vi "identifyPortTypeWithFirstByte_2.vi"(1 "input_str":string) -> (0 "show_str_portType":string)   [LabVIEW 2011]
panel:
  # "本VI已经验证过下列对应关系        OK\nhex  decimal  portType\n03    3           SFP+\n\n11    17          QSFP+\n0D    13         QSFP+\n\n0F     15         HD\n10     16         HD\n14     20         HD\n15     21         HD"
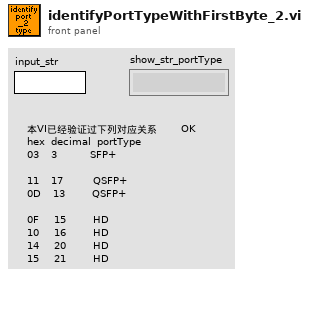
[diagram p1: front panel]
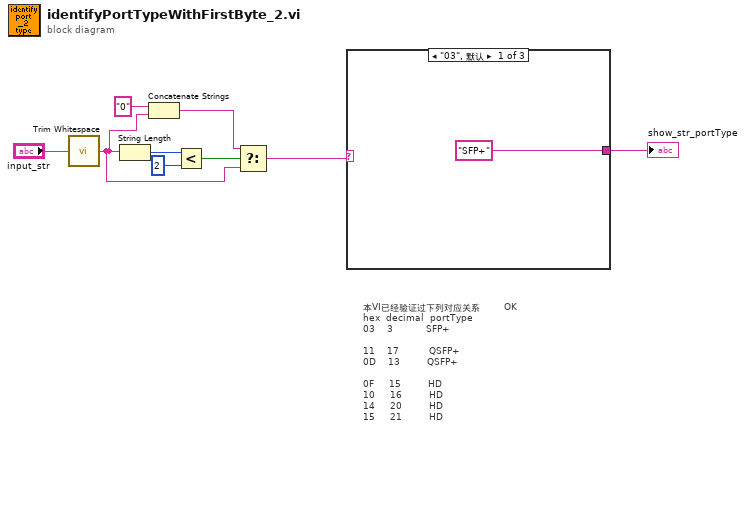
[diagram p0: block diagram]
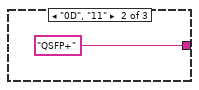
[diagram p2: hidden frame]
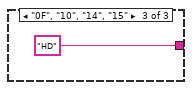
[diagram p3: hidden frame]
diagram:
  # "本VI已经验证过下列对应关系        OK\nhex  decimal  portType\n03    3           SFP+\n\n11    17          QSFP+\n0D    13         QSFP+\n\n0F     15         HD\n10     16         HD\n14     20         HD\n15     21         HD"
  n1 = call <vilib>:"Trim Whitespace.vi"("string"="input_str") -> ("trimmed string"=w2:string)  [unwired: 1 in]
  n2 = String Length(string=w2) -> (length=w7:i32)
  n3 = Concatenate Strings("0" ("字符串"), w2) -> (w3:string)
  n4 = Less?(x=w7, y=2) -> (x < y?=w5:bool)
  n5 = Select(t=w3, s=w5, f=w2) -> (s? t:f=w1:string)
  n6 = case shown="\"03\", 默认" w1 {
    tunnel: ["SFP+" "QSFP+" "HD"] -> w9
    frame "03", Default {
    }
    frame "0D", "11" {
    }
    frame "0F", "10", "14", "15" {
    }
  }
  "show_str_portType" <- w9
